vi "test_libssh2_sftp_rename.vi"() -> ()   [LabVIEW 2013, in "libssh2_integration_tests.lvlib"]
uses:
  libssh2_integration_tests.lvlib
  <vilib>/addons/_JKI Toolkits/Caraya/classes/Test/Test.lvclass
  <vilib>/addons/_JKI Toolkits/Caraya/classes/Assert/Assert.lvclass
  libssh2/libssh2.lvlib
panel:
  out "error out":errorcluster
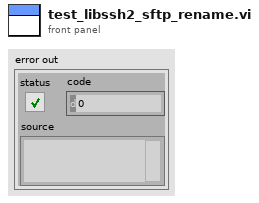
[diagram p1: front panel]
types:
  T1 = typedef "libssh2.lvlib/Session Refnum.ctl" = refnum<k1>
  T2 = typedef "libssh2.lvlib/SFTP Refnum.ctl" = refnum<k1>
  T3 = typedef "libssh2.lvlib/SFTP Handle Refnum.ctl" = refnum<k1>
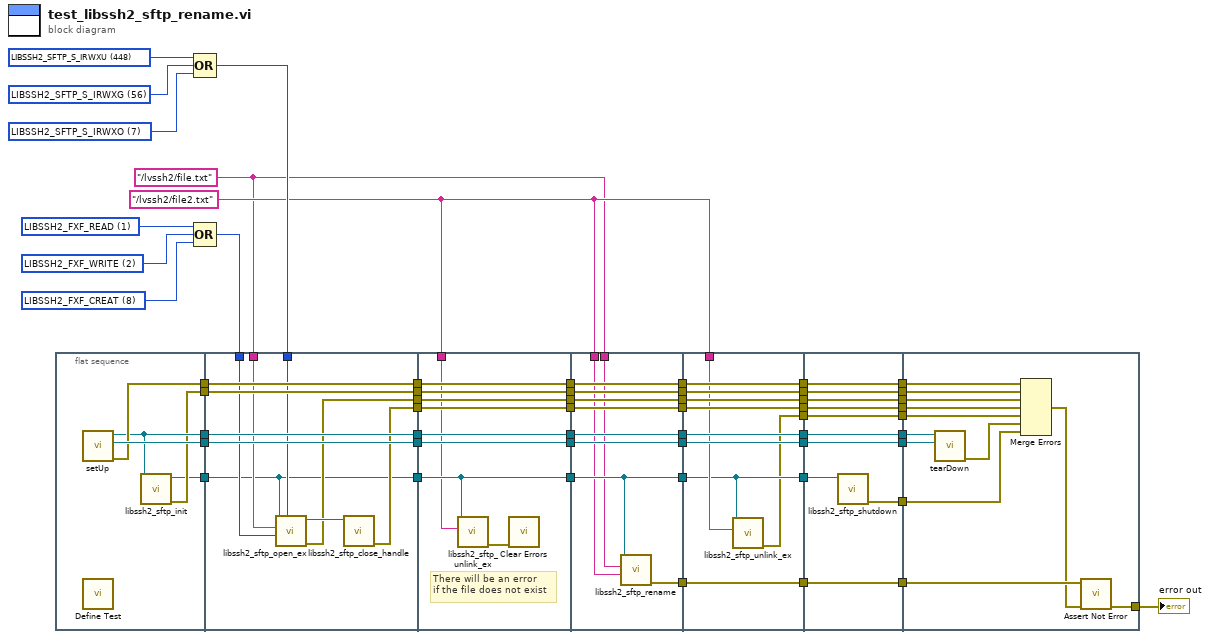
[diagram p0: block diagram]
diagram:
  w4 = "/lvssh2/file2.txt" ("filename")
  w45 = u32 2 items=["LIBSSH2_FXF_READ"=1, "LIBSSH2_FXF_WRITE"=2, "LIBSSH2_FXF_APPEND"=4, "LIBSSH2_FXF_CREAT"=8, "LIBSSH2_FXF_TRUNC"=16, "LIBSSH2_FXF_EXCL"=32] ("flags")
  w46 = u32 1 items=["LIBSSH2_FXF_READ"=1, "LIBSSH2_FXF_WRITE"=2, "LIBSSH2_FXF_APPEND"=4, "LIBSSH2_FXF_CREAT"=8, "LIBSSH2_FXF_TRUNC"=16, "LIBSSH2_FXF_EXCL"=32] ("flags")
  w44 = u32 8 items=["LIBSSH2_FXF_READ"=1, "LIBSSH2_FXF_WRITE"=2, "LIBSSH2_FXF_APPEND"=4, "LIBSSH2_FXF_CREAT"=8, "LIBSSH2_FXF_TRUNC"=16, "LIBSSH2_FXF_EXCL"=32] ("flags")
  w3 = "/lvssh2/file.txt" ("filename")
  w48 = 7 items=["LIBSSH2_SFTP_S_IRWXU"=448, "LIBSSH2_SFTP_S_IRUSR"=256, "LIBSSH2_SFTP_S_IWUSR"=128, "LIBSSH2_SFTP_S_IXUSR"=64, "LIBSSH2_SFTP_S_IRWXG"=56, "LIBSSH2_SFTP_S_IRGRP"=32, "LIBSSH2_SFTP_S_IWGRP"=16, "LIBSSH2_SFTP_S_IXGRP"=8, "LIBSSH2_SFTP_S_IRWXO"=7, "LIBSSH2_SFTP_S_IROTH"=4, "LIBSSH2_SFTP_S_IWOTH"=2, "LIBSSH2_SFTP_S_IXOTH"=1] ("mode")
  w49 = 56 items=["LIBSSH2_SFTP_S_IRWXU"=448, "LIBSSH2_SFTP_S_IRUSR"=256, "LIBSSH2_SFTP_S_IWUSR"=128, "LIBSSH2_SFTP_S_IXUSR"=64, "LIBSSH2_SFTP_S_IRWXG"=56, "LIBSSH2_SFTP_S_IRGRP"=32, "LIBSSH2_SFTP_S_IWGRP"=16, "LIBSSH2_SFTP_S_IXGRP"=8, "LIBSSH2_SFTP_S_IRWXO"=7, "LIBSSH2_SFTP_S_IROTH"=4, "LIBSSH2_SFTP_S_IWOTH"=2, "LIBSSH2_SFTP_S_IXOTH"=1] ("mode")
  w50 = 448 items=["LIBSSH2_SFTP_S_IRWXU"=448, "LIBSSH2_SFTP_S_IRUSR"=256, "LIBSSH2_SFTP_S_IWUSR"=128, "LIBSSH2_SFTP_S_IXUSR"=64, "LIBSSH2_SFTP_S_IRWXG"=56, "LIBSSH2_SFTP_S_IRGRP"=32, "LIBSSH2_SFTP_S_IWGRP"=16, "LIBSSH2_SFTP_S_IXGRP"=8, "LIBSSH2_SFTP_S_IRWXO"=7, "LIBSSH2_SFTP_S_IROTH"=4, "LIBSSH2_SFTP_S_IWOTH"=2, "LIBSSH2_SFTP_S_IXOTH"=1] ("mode")
  n1 = flat-sequence {
    tunnel: [w59] -> w56
    tunnel: [w61] -> w55
    tunnel: [w60] -> w54
    tunnel: [w58] -> w52
    tunnel: [w57] -> w51
    tunnel: w56 -> [w72]
    tunnel: w55 -> [w71]
    tunnel: [w72] -> w34
    tunnel: [w71] -> w32
    tunnel: [w62] -> w30
    tunnel: [w70] -> w28
    tunnel: w54 -> [w70]
    tunnel: w52 -> [w69]
    tunnel: [w69] -> w26
    tunnel: w51 -> [w62]
    tunnel: w47 -> [w68]
    tunnel: w3 -> [w67]
    tunnel: w43 -> [w66]
    tunnel: [w64] -> w24
    tunnel: [w63] -> w22
    tunnel: w34 -> [w81]
    tunnel: [w81] -> w33
    tunnel: w32 -> [w80]
    tunnel: [w80] -> w31
    tunnel: w30 -> [w74]
    tunnel: [w74] -> w29
    tunnel: w28 -> [w79]
    tunnel: [w79] -> w27
    tunnel: w26 -> [w78]
    tunnel: [w78] -> w25
    tunnel: w24 -> [w77]
    tunnel: [w77] -> w23
    tunnel: w22 -> [w76]
    tunnel: [w76] -> w21
    tunnel: w4 -> [w73]
    tunnel: w33 -> [w91]
    tunnel: [w91] -> w20
    tunnel: w31 -> [w90]
    tunnel: [w90] -> w18
    tunnel: w29 -> [w85]
    tunnel: [w85] -> w16
    tunnel: [w84] -> w14
    tunnel: w27 -> [w89]
    tunnel: [w89] -> w12
    tunnel: w25 -> [w88]
    tunnel: [w88] -> w10
    tunnel: [w87] -> w8
    tunnel: w23 -> [w87]
    tunnel: w21 -> [w86]
    tunnel: [w86] -> w6
    tunnel: w3 -> [w83]
    tunnel: w4 -> [w82]
    tunnel: w20 -> [w101]
    tunnel: [w101] -> w19
    tunnel: w18 -> [w100]
    tunnel: [w100] -> w17
    tunnel: w16 -> [w93]
    tunnel: [w93] -> w15
    tunnel: w14 -> [w99]
    tunnel: [w99] -> w13
    tunnel: w12 -> [w98]
    tunnel: [w98] -> w11
    tunnel: w10 -> [w97]
    tunnel: [w97] -> w9
    tunnel: w8 -> [w96]
    tunnel: [w96] -> w7
    tunnel: w6 -> [w95]
    tunnel: [w95] -> w5
    tunnel: w4 -> [w94]
    tunnel: [w92] -> w2
    tunnel: w19 -> [w111]
    tunnel: [w111] -> w42
    tunnel: w17 -> [w110]
    tunnel: [w110] -> w41
    tunnel: w15 -> [w106]
    tunnel: w13 -> [w109]
    tunnel: [w109] -> w40
    tunnel: w11 -> [w108]
    tunnel: [w108] -> w39
    tunnel: w9 -> [w107]
    tunnel: [w107] -> w38
    tunnel: [w105] -> w37
    tunnel: w7 -> [w104]
    tunnel: [w104] -> w36
    tunnel: w5 -> [w103]
    tunnel: [w103] -> w35
    tunnel: w2 -> [w102]
    tunnel: [w102] -> w1
    tunnel: w42 -> [w123]
    tunnel: w41 -> [w122]
    tunnel: w40 -> [w121]
    tunnel: w39 -> [w120]
    tunnel: [w117] -> w53
    tunnel: w38 -> [w116]
    tunnel: w37 -> [w115]
    tunnel: w36 -> [w114]
    tunnel: w35 -> [w113]
    tunnel: w1 -> [w112]
    frame #0 {
      n2 = call "setUp.vi"() -> ("error out"=w60:errorcluster, "connection ID"=w61:refnum<k5>, "session"=w59:T1)  [unwired: 9 in]
      n3 = call <vilib>:"Define Test.vi"() -> ()  [unwired: 10 in, 2 out]
      n4 = call "libssh2_sftp_init.vi"("session"=w59) -> ("error out"=w58:errorcluster, "sftp"=w57:T2)  [unwired: 9 in]
    }
    frame #1 {
      n5 = call "libssh2_sftp_open_ex.vi"("mode"=w68, "flags"=w66, "filename"=w67, "sftp"=w62) -> ("error out"=w64:errorcluster, "sftp handle"=w65:T3)  [unwired: 6 in]
      n6 = call "libssh2_sftp_close_handle.vi"("sftp handle"=w65) -> ("error out"=w63:errorcluster)  [unwired: 10 in]
    }
    frame #2 {
      # "There will be an error\nif the file does not exist"
      n7 = call "libssh2_sftp_unlink_ex.vi"("file"=w73, "sftp"=w74) -> ("error out"=w75:errorcluster)  [unwired: 9 in]
      n8 = call <vilib>:"Clear Errors.vi"("error in (no error)"=w75) -> ()  [unwired: 6 in, 1 out]
    }
    frame #3 {
      n9 = call "libssh2_sftp_rename.vi"("destination file"=w82, "source file"=w83, "sftp"=w85) -> ("error out"=w84:errorcluster)  [unwired: 8 in]
    }
    frame #4 {
      n10 = call "libssh2_sftp_unlink_ex.vi"("file"=w94, "sftp"=w93) -> ("error out"=w92:errorcluster)  [unwired: 9 in]
    }
    frame #5 {
      n11 = call "libssh2_sftp_shutdown.vi"("sftp"=w106) -> ("error out"=w105:errorcluster)  [unwired: 10 in]
    }
    frame #6 {
      n12 = call "tearDown.vi"("connection ID"=w122, "session"=w123) -> ("error out"=w119:errorcluster)  [unwired: 9 in]
      n13 = Merge Errors(w120, w116, w114, w113, w112, w119, w115) -> (w118:errorcluster)
      n14 = call <vilib>:"Assert Not Error.vi"("error in (no error)"=w118, "Not Error?"=w121) -> ("error out"=w117:errorcluster)  [unwired: 8 in, 1 out]
    }
  }
  n15 = Compound Arithmetic op=OR(w50, w49, w48) -> (w47:i32)
  n16 = Compound Arithmetic op=OR(w46, w45, w44) -> (w43:u32)
  "error out" <- w53
